vi "Write data file.vi"(8 "error in (no error)":errorcluster, 9 "Data in Volts":i16[](array[numeric]), 10 "Path":path) -> (0 "error out":errorcluster)   [LabVIEW 2015, in "Gage digitizer actor.lvclass"]
uses:
  Gage digitizer actor.lvclass
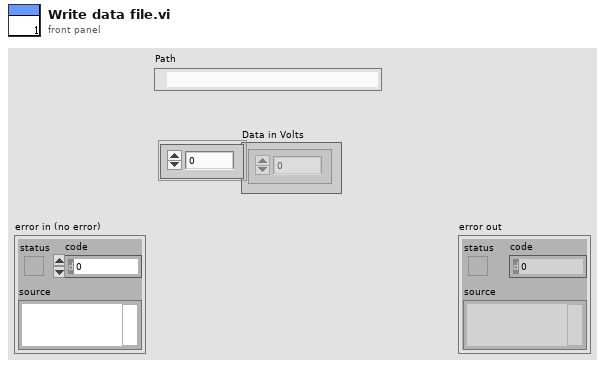
[diagram p1: front panel]
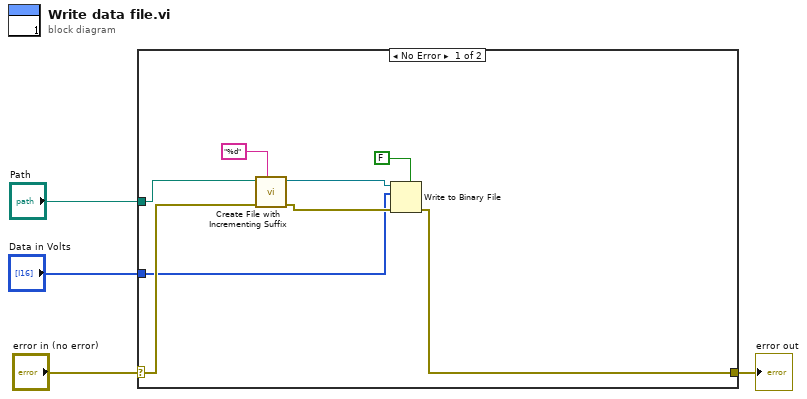
[diagram p0: block diagram]
diagram:
  n1 = case shown="No Error" "error in (no error)" {
    selector: "error in (no error)" -> [w11 w13]
    tunnel: [w6 w13] -> w3
    tunnel: "Path" -> [w12 _]
    tunnel: "Data in Volts" -> [w5 _]
    frame No Error {
      n2 = call <vilib>:"Create File with Incrementing Suffix.vi"("format string (\" (%d)\")"="%d" ("format string (\" (%d)\")"), "error in (no error)"=w11, "file path"=w12) -> ("error out"=w7:errorcluster, "refnum out"=w9:refnum<file>)  [unwired: 6 in, 1 out]
      n3 = Write to Binary File(file (use dialog)=w9, data=w5, error in=w7, 5:FALSE ("prepend array or string size? (T)")) -> (error out=w6:errorcluster)  [unwired: 2 in, 2 out]
    }
    frame Error {
    }
  }
  "error out" <- w3
